vi "Drive_Utils_CalculateScale.vi"(3 "error in":errorcluster, 4 "Right distance":dbl, 5 "Left distance":dbl) -> (0 "error out":errorcluster, 1 "Right scale":dbl=1.0, 2 "Left scale":dbl=1.0)   [LabVIEW 2009, in "Drive.lvlib" / "Drive_Utils.lvlib"]
doc: "This VI calculates the scale factor for left and right side of the robot based on the distances. This factor is used in calculate in CalculateSpeed VI to synchronize movements of both sides."
uses:
  Drive_Utils.lvlib
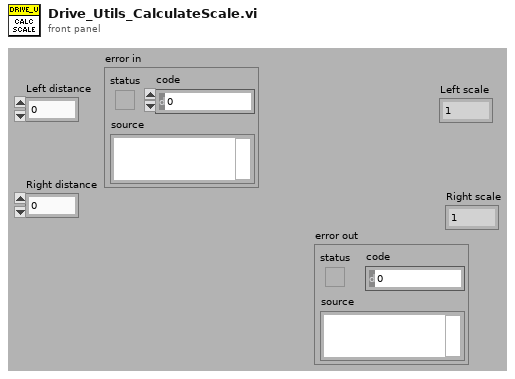
[diagram p1: front panel]
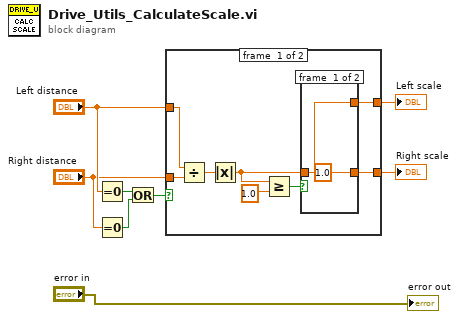
[diagram p0: block diagram]
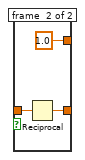
[diagram p2: hidden frame]
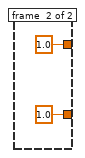
[diagram p3: hidden frame]
diagram:
  n1 = Equal To 0?(x="Left distance") -> (x = 0?=w8:bool)
  n2 = Equal To 0?(x="Right distance") -> (x = 0?=w7:bool)
  n3 = Or(x=w8, y=w7) -> (x .or. y?=w6:bool)
  n4 = case shown="False" w6 {
    tunnel: [w10 1.0 ("Left scale")] -> w5
    tunnel: [w9 1.0 ("Left scale")] -> w4
    tunnel: "Left distance" -> [w16 _]
    tunnel: "Right distance" -> [w15 _]
    frame #0 {
      n5 = Divide(x=w16, y=w15) -> (x/y=w14:dbl)
      n6 = Absolute Value(x=w14) -> (abs(x)=w11:dbl)
      n7 = Greater Or Equal?(x=w11, y=1.0) -> (x >= y?=w13:bool)
      n8 = case shown="False" w13 {
        tunnel: w11 -> [w17 w20]
        tunnel: [w17 1.0] -> w10
        tunnel: [1.0 w19] -> w9
        frame #0 {
        }
        frame #1 {
          n9 = Reciprocal(x=w20) -> (1/x=w19:dbl)
        }
      }
    }
    frame #1 {
    }
  }
  "Left scale" <- w5
  "Right scale" <- w4
  "error out" <- "error in"
